vi "Actor Core.vi"(8 "Error In":errorcluster, 11 "Core In":refnum<class "Core.lvclass">) -> (0 "Error Out":errorcluster, 3 "Actor Out":refnum<class "Actor.lvclass">)   [LabVIEW 2019, in "Core.lvlib" / "Core.lvclass"]
doc: "(<B>Filename</B>: Actor Framework.lvlib:Actor.lvclass:Actor Core.vi)\n\nReceives messages to the actor, reacts to them, and initiates any error handling that may shut the actor down.\n\nDescendant classes may override this VI to append parallel tasks for the actor to complete while it handles messages. Overrides use the Call Parent Method node."
uses:
  Core.lvclass
  C:/Projekty/_Poboczne/PC_ActorFramework/07_Program/LABVIEW/02_Source/Modules/ModuleAbstract/ModuleAbstract/ModuleAbstract.lvclass
  C:/Program Files (x86)/National Instruments/LabVIEW 2019/vi.lib/ActorFramework/Actor/Actor.lvclass
  <vilib>/ActorFramework/Actor/Actor.lvclass
  ModuleAbstract/ModuleAbstract/ModuleAbstract.lvclass/ModuleAbstract.ctl
  ModuleAbstract/ModuleAbstract/ModuleAbstract.lvclass
  <vilib>/ActorFramework/Stop Msg/Stop Msg.lvclass
panel:
  in  "Stop":bool
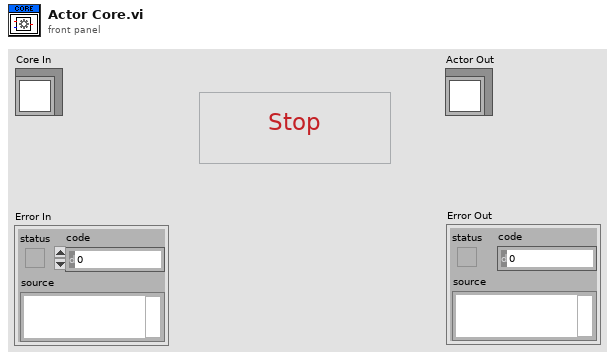
[diagram p1: front panel]
types:
  T1 = enum32{"Invalid", "Standard", "Closed", "Hidden", "Minimized", "Maximized"}
  T2 = cluster{"EventLog":cluster{"REF":refnum<class "EventLog.lvclass">}}
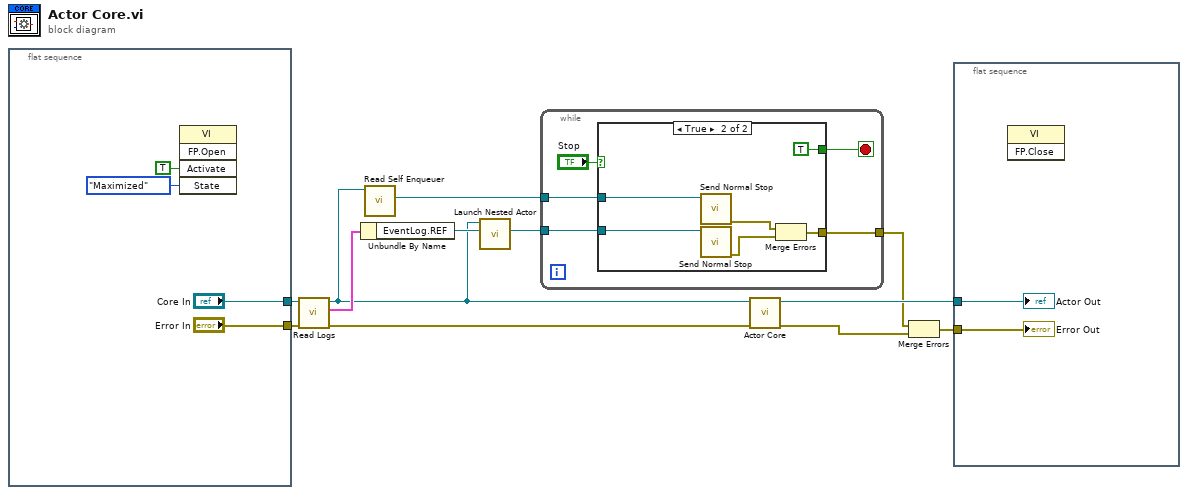
[diagram p0: block diagram]
diagram:
  n1 = flat-sequence {
    tunnel: ["Error In"] -> w6
    tunnel: ["Core In"] -> w11
    frame #0 {
      n2 = invoke class="VI" method="FP.Open"("Activate"=TRUE ("Activate?"), "State"=T1."Maximized") -> ()  [unwired: 3 in, 5 out]
    }
  }
  n3 = call "Read Logs.vi"("error in (no error)"=w6, "ModuleAbstract in"=w11) -> ("error out"=w5:errorcluster, "Logs"=w8:T2, "ModuleAbstract out"=w4:refnum<class "Core.lvclass">)  [unwired: 7 in]
  n4 = Unbundle By Name(w8) -> ("EventLog.REF"=w7:refnum<class "EventLog.lvclass">)
  n5 = call <vilib>:"Read Self Enqueuer.vi"("Actor"=w4) -> ("Self Enqueuer"=w3:refnum<class "Message Enqueuer.lvclass">)  [unwired: 10 in]
  n6 = call <vilib>:"Launch Nested Actor.vi"("Nested Actor"=w7, "Caller Actor in"=w4) -> ("Nested Actor's Enqueuer"=w2:refnum<class "Message Enqueuer.lvclass">)  [unwired: 7 in, 2 out]
  n7 = while {
    tunnel: w3 -> [w20]
    tunnel: w2 -> [w18]
    tunnel: [w17] -> w1
    stop <- w19 stop-if-true
    n8 = case shown="True" "Stop" {
      tunnel: w20 -> [_ w27]
      tunnel: [_ TRUE] -> w19
      tunnel: w18 -> [_ w25]
      tunnel: [_ w22] -> w17
      frame False {
      }
      frame True {
        n9 = call <vilib>:"Send Normal Stop.vi"("Message Enqueuer"=w27) -> ("error out"=w23:errorcluster)  [unwired: 10 in]
        n10 = call <vilib>:"Send Normal Stop.vi"("Message Enqueuer"=w25) -> ("error out"=w24:errorcluster)  [unwired: 10 in]
        n11 = Merge Errors(w23, w24) -> (w22:errorcluster)
      }
    }
  }
  n12 = call-parent "Actor Core.vi"("error in"=w5, "Actor in"=w4) -> ("error out"=w9:errorcluster, "Actor out"=w12:refnum<class "Actor.lvclass">)  [unwired: 8 in]
  n13 = Merge Errors(w1, w9) -> (w10:errorcluster)
  n14 = flat-sequence {
    tunnel: w12 -> [w29]
    tunnel: w10 -> [w28]
    frame #0 {
      n15 = invoke class="VI" method="FP.Close"() -> ()  [unwired: 3 in, 3 out]
      "Error Out" <- w28
      "Actor Out" <- w29
    }
  }
